vi "CPP_ProjNumToPrefGlob.vi"() -> ()   [LabVIEW 2010]
uses:
  Globals/Preference_global.vi
panel:
  out "NewProjectNumber":string
  out "OriginalProjectNumber":string
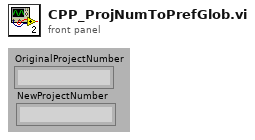
[diagram p1: front panel]
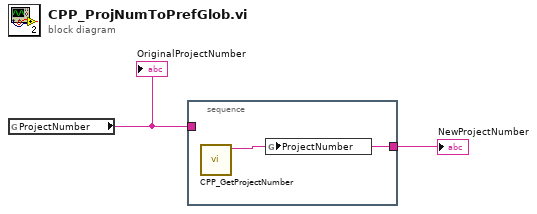
[diagram p0: block diagram]
diagram:
  n1 = global read "Preference_global.vi" "ProjectNumber"() -> (w2:string)
  "OriginalProjectNumber" <- w2
  n2 = stacked-sequence {
    tunnel: w2 -> [_]
    tunnel: [w3] -> w1
    frame #0 {
      n3 = call "CPP_GetProjectNumber.vi"() -> ("ProjectNumber"=w3:string)  [unwired: 11 in]
      n4 = global write "Preference_global.vi" "ProjectNumber"(w3) -> ()
    }
  }
  "NewProjectNumber" <- w1
